vi "Run or Halt Fan.vi"(8 "error in (no error)":errorcluster, 10 "Running?":bool=TRUE, 11 "Dual Fan in":refnum<class "Dual Fan.lvclass">) -> (0 "error out":errorcluster, 3 "Dual Fan out":refnum<class "Dual Fan.lvclass">)   [LabVIEW 2025, in "Dual Fan.lvlib" / "Dual Fan.lvclass"]
doc: "Call this method to tell the fans to start or stop."
uses:
  Dual Fan.lvclass
  Dual Fan.lvclass/Dual Fan.ctl
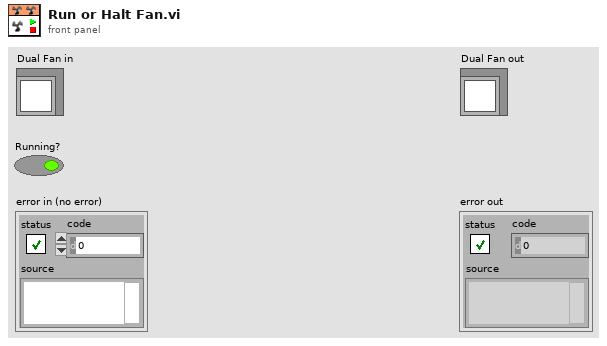
[diagram p1: front panel]
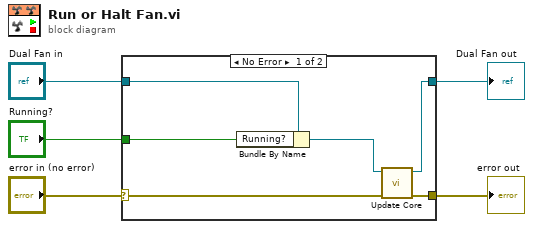
[diagram p0: block diagram]
diagram:
  n1 = case shown="No Error" "error in (no error)" {
    selector: "error in (no error)" -> [w7 w13]
    tunnel: [w8 w13] -> w4
    tunnel: [w9 w12] -> w2
    tunnel: "Dual Fan in" -> [w11 w12]
    tunnel: "Running?" -> [w6 _]
    frame No Error {
      n2 = Bundle By Name(cluster=w11, "Running?"=w6) -> (w10:refnum<class "Dual Fan.lvclass">)
      n3 = call-dynamic "Update Core.vi"("error in (no error)"=w7, "Dual Fan in"=w10) -> ("error out"=w8:errorcluster, "Dual Fan out"=w9:refnum<class "Dual Fan.lvclass">)  [unwired: 8 in]
    }
    frame Error {
    }
  }
  "error out" <- w4
  "Dual Fan out" <- w2
